vi "calibrate ESR.vi"(7 "Processing loop variables":T1 {"CurrInverter"."last updated" format="%<%H:%M\n%d/%m/%Y>T"; "CurrInverter"."set flag" items=["False", "True"]}, 8 "error in (no error)":errorcluster, 9 "Max ESR":dbl[](array[numeric]), 11 "Acquisition mode in":T8) -> (0 "error out":errorcluster, 3 "Processing loop vars out":T1 {"CurrInverter"."last updated" format="%<%H:%M\n%d/%m/%Y>T"; "CurrInverter"."set flag" items=["False", "True"]})   [LabVIEW 2019, in "Main.lvclass"]
uses:
  Main.lvclass
  Common/DataTypes/Acquisition Mode--cluster.ctl
  DataTypes/averaging variables.ctl
  DataTypes/ESR alarm variables.ctl
  Common/DataTypes/inverter gain range--cluster.ctl
  Common/DataTypes/inverter offset range--cluster.ctl
  Common/DataTypes/inverter info v2--cluster.ctl
  Common/DataTypes/Inverter database record v2--cluster.ctl
  DataTypes/Processing loop variables--cluster.ctl
panel:
  out "Calibration":dbl
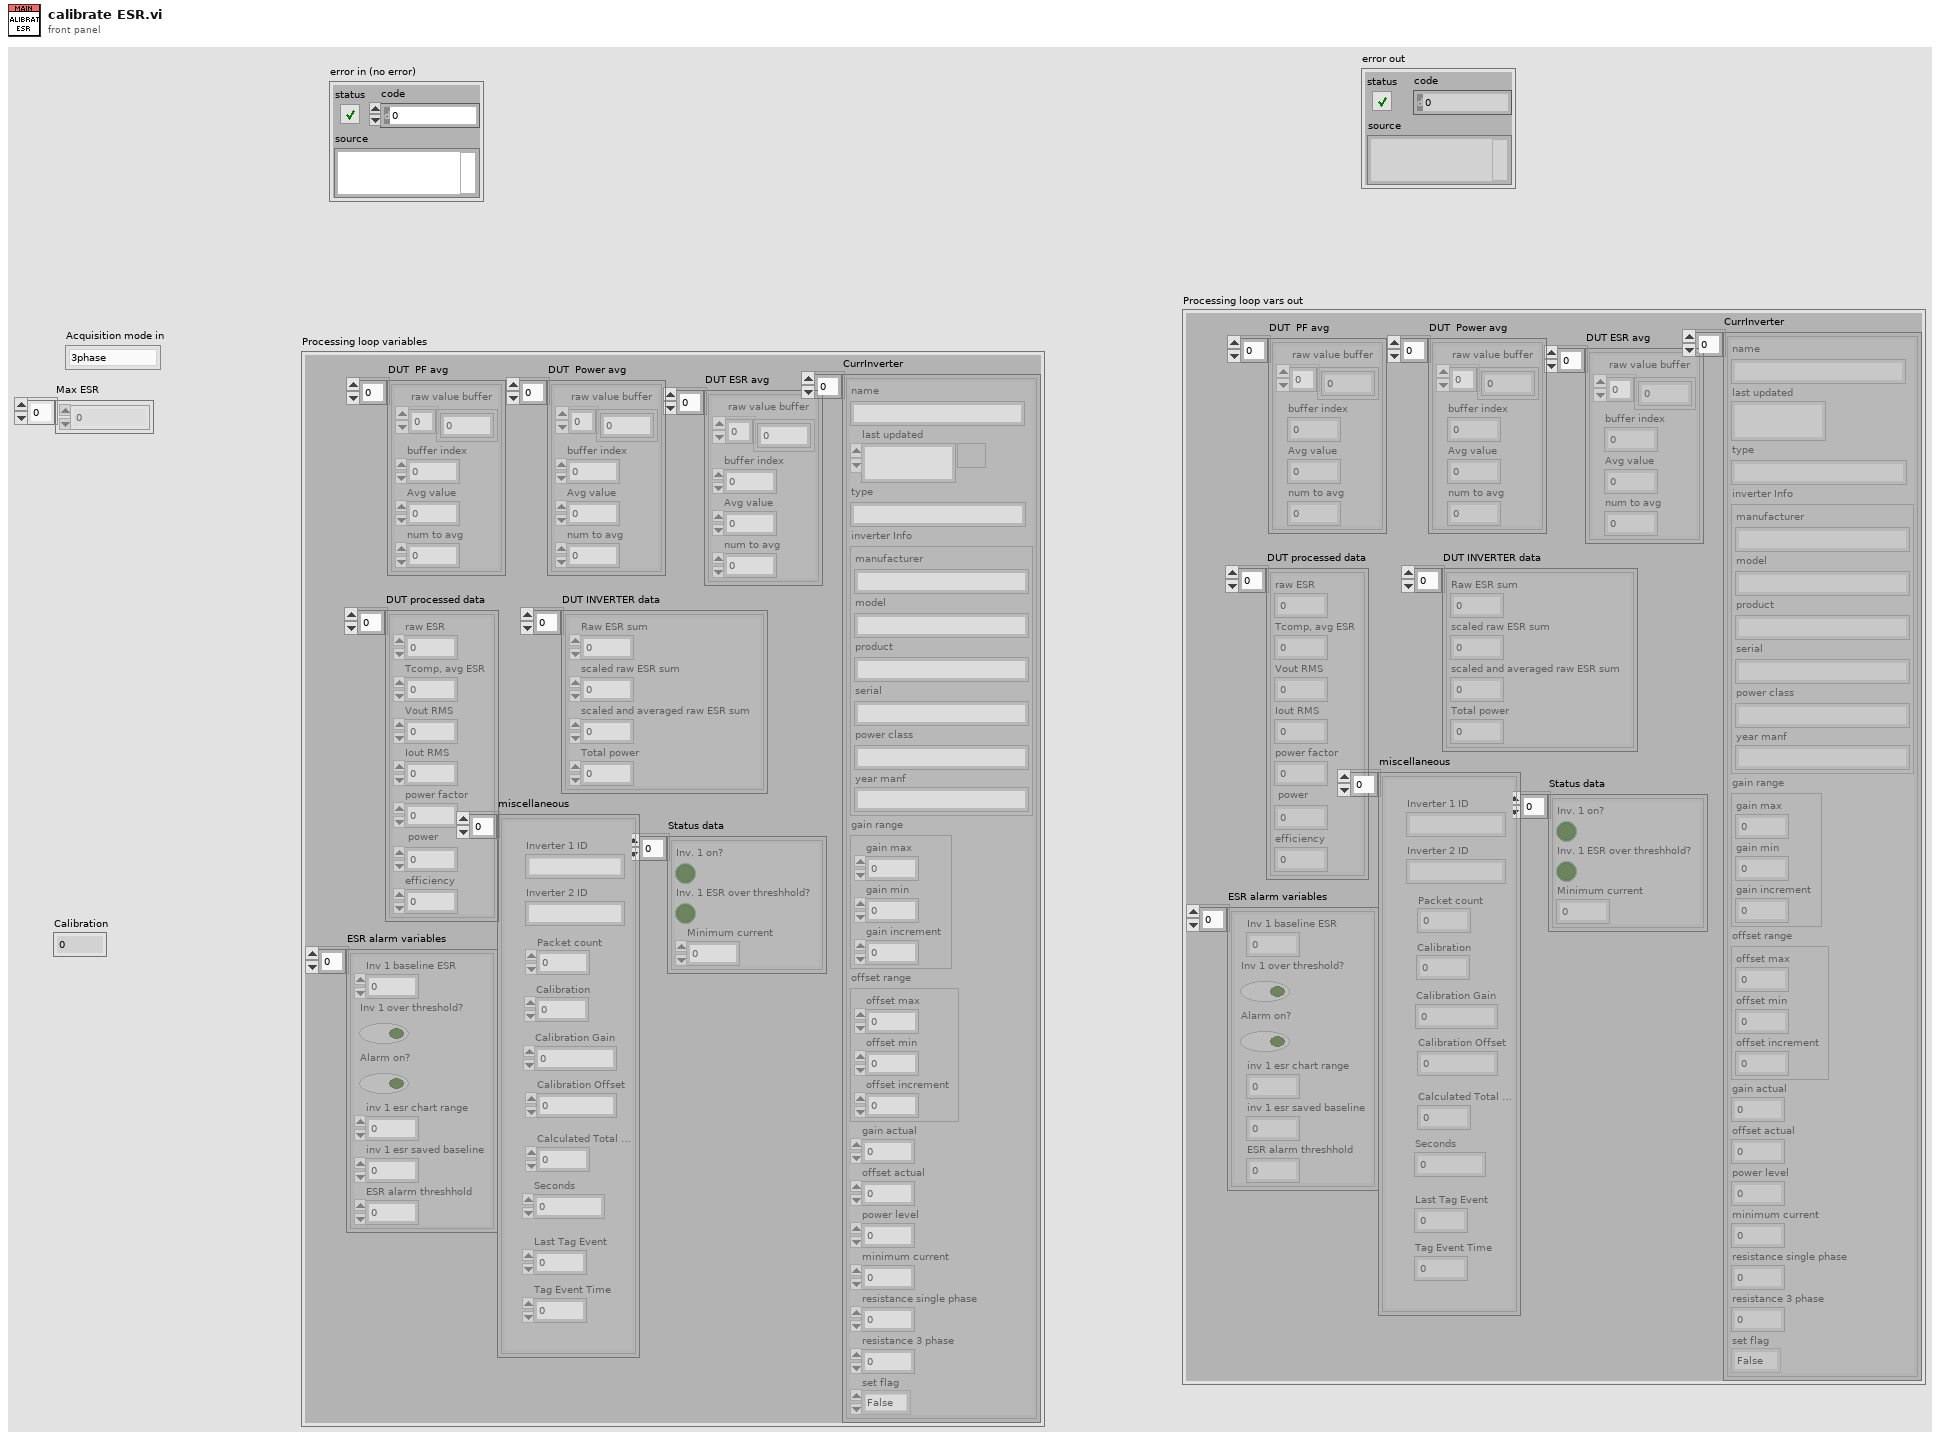
[diagram p1: front panel]
types:
  T1 = typedef "Main.lvclass/Processing loop variables--cluster.ctl" = cluster{"DUT ESR avg":T2[], "DUT  PF avg":T2[], "DUT  Power avg ":T2[], "DUT processed data":cluster{"raw ESR":dbl, "Tcomp, avg ESR":dbl, "Vout RMS":dbl, "Iout RMS":dbl, "power factor":dbl, "power":dbl, "efficiency":dbl}[], "ESR alarm variables":T3[], "Status data":cluster{"Inv. 1 on?":bool, "Inv. 1 ESR over threshhold?":bool, "Minimum current":dbl}[], "CurrInverter":T4[], "miscellaneous":cluster{"Inverter 1 ID":string, "Inverter 2 ID":string, "Packet count":u32, "Calibration":dbl, "Calibration Gain":dbl, "Calibration Offset":dbl, "Calculated Total Power":dbl, "Seconds":dbl, "Last Tag Event":dbl, "Tag Event Time":dbl}[], "DUT INVERTER data":cluster{"Raw ESR sum":dbl, "scaled raw ESR sum":dbl, "scaled and averaged raw ESR sum":dbl, "Total power":dbl}[]}
  T2 = typedef "Main.lvclass/averaging variables.ctl" = cluster{"raw value buffer":dbl[], "buffer index":i32, "Avg value":dbl, "num to avg":i32}
  T3 = typedef "Main.lvclass/ESR alarm variables.ctl" = cluster{"Inv 1 baseline ESR":dbl, "Inv 1 over threshold?":bool, "Alarm on?":bool, "inv 1 esr chart range":dbl, "inv 1 esr saved baseline":dbl, "ESR alarm threshhold":dbl}
  T4 = typedef "Inverter database record v2--cluster.ctl" = cluster{"name":string, "last updated":timestamp, "type":string, "inverter Info":T5, "gain range":T6, "offset range":T7, "gain actual":dbl, "offset actual":dbl, "power level":dbl, "minimum current":dbl, "resistance single phase":dbl, "resistance 3 phase":dbl, "set flag":u16}
  T5 = typedef "inverter info v2--cluster.ctl" = cluster{"manufacturer":string, "model":string, "product":string, "serial":string, "power class":string, "year manf":string}
  T6 = typedef "inverter gain range--cluster.ctl" = cluster{"gain max":dbl, "gain min":dbl, "gain increment":dbl}
  T7 = typedef "inverter offset range--cluster.ctl" = cluster{"offset max":dbl, "offset min":dbl, "offset increment":dbl}
  T8 = typedef "Acquisition Mode--cluster.ctl" = enum16{"3phase", "Single"}
  T9 = cluster{"Inverter 1 ID":string, "Inverter 2 ID":string, "Packet count":u32, "Calibration":dbl, "Calibration Gain":dbl, "Calibration Offset":dbl, "Calculated Total Power":dbl, "Seconds":dbl, "Last Tag Event":dbl, "Tag Event Time":dbl}[]
  T10 = cluster{"Raw ESR sum":dbl, "scaled raw ESR sum":dbl, "scaled and averaged raw ESR sum":dbl, "Total power":dbl}[]
  T11 = cluster{"Inverter 1 ID":string, "Inverter 2 ID":string, "Packet count":u32, "Calibration":dbl, "Calibration Gain":dbl, "Calibration Offset":dbl, "Calculated Total Power":dbl, "Seconds":dbl, "Last Tag Event":dbl, "Tag Event Time":dbl}
  T12 = cluster{string, "time string":string, "t":dbl, "Calibration Gain":dbl, "Calibration Offset":dbl, "Max ESR":dbl, "Acquisition mode in":T8, "name":string, "serial":string, "Total power":dbl}
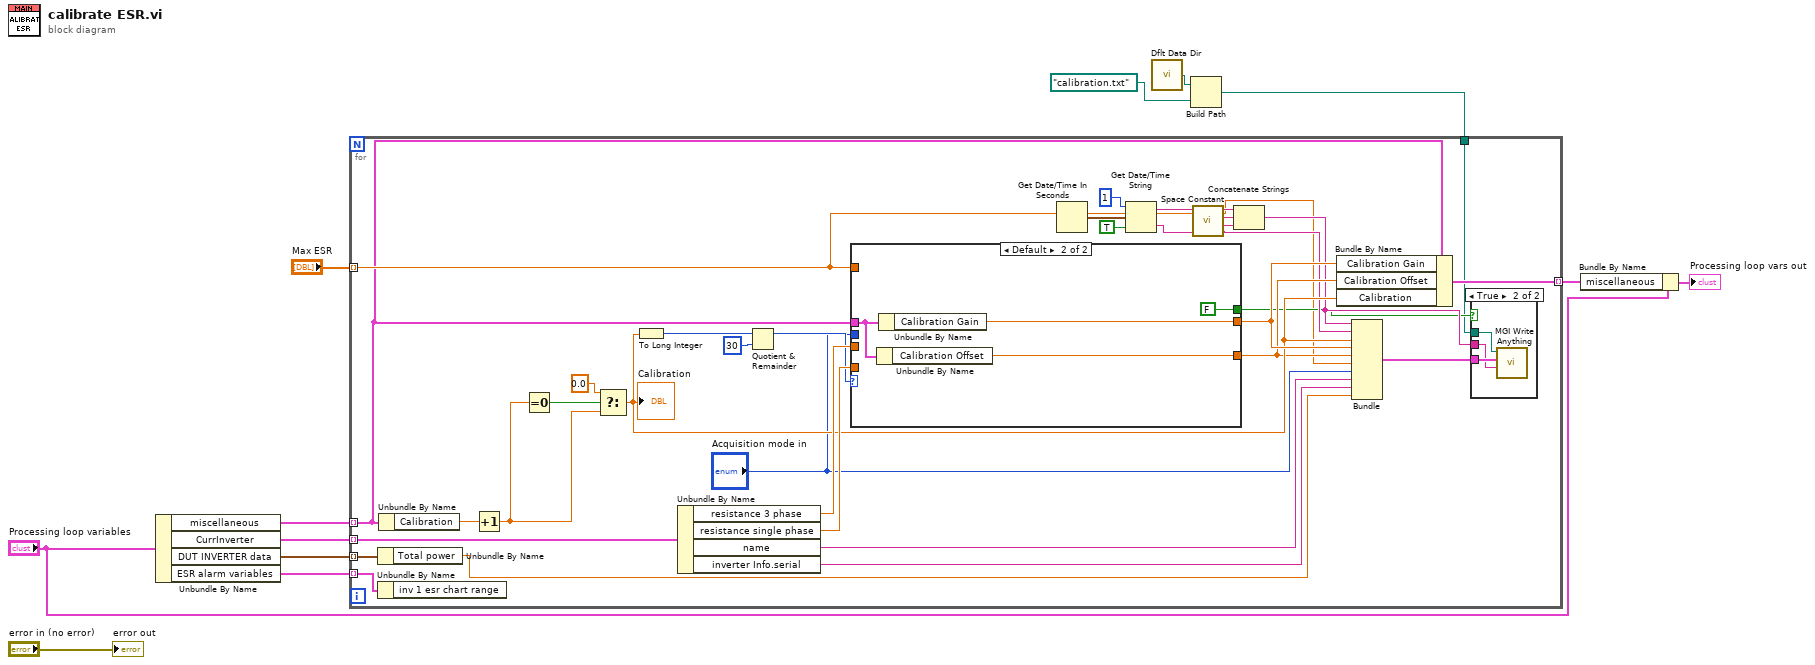
[diagram p0: block diagram]
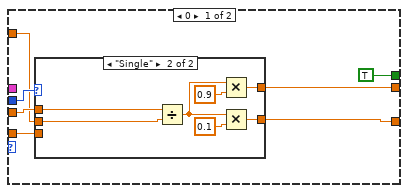
[diagram p3: hidden frame]
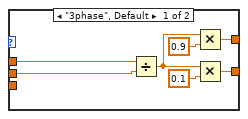
[diagram p4: hidden frame]
diagram:
  n1 = Unbundle By Name("Processing loop variables") -> ("miscellaneous"=w11:T9, "CurrInverter"=w10:T4[], "DUT INVERTER data"=w9:T10, "ESR alarm variables"=w5:T3[])
  n2 = call <vilib>:"Dflt Data Dir.vi"() -> ("App:Default Data Directory"=w3:path)
  n3 = Build Path(base path=w3, name or relative path=path "calibration.txt") -> (appended path=w1:path)
  n4 = for {
    tunnel: w11 -> [w14] mode=indexing
    tunnel: w10 -> [w44] mode=indexing
    tunnel: w9 -> [w43] mode=indexing
    tunnel: [w42] -> w6 mode=indexing
    tunnel: w5 -> [w16] mode=indexing
    tunnel: "Max ESR" -> [w15] mode=indexing
    tunnel: w1 -> [w13]
    n5 = Unbundle By Name(w43) -> ("Total power"=w17:dbl)
    n6 = Unbundle By Name(w16) -> ()  [unwired: 1 out]
    n7 = Unbundle By Name(w14) -> ("Calibration"=w40:dbl)
    n8 = Increment(x=w40) -> (x+1=w36:dbl)
    n9 = Equal To 0?(x=w36) -> (x = 0?=w34:bool)
    n10 = Select(t=0.0, s=w34, f=w36) -> (s? t:f=w30:dbl)
    "Calibration" <- w30
    n11 = To Long Integer(number=w30) -> (32bit integer=w32:i32)
    n12 = Unbundle By Name(w44) -> ("resistance 3 phase"=w41:dbl, "resistance single phase"=w39:dbl, "name"=w22:string, "inverter Info.serial"=w21:string)
    n13 = Quotient & Remainder(x=w32, y=30) -> (x-y*floor(x/y)=w31:i32)  [unwired: 1 out]
    n14 = case shown="Default" w31 {
      tunnel: "Acquisition mode in" -> [w54 _]
      tunnel: w41 -> [w53 _]
      tunnel: w15 -> [w52 _]
      tunnel: w39 -> [w51 _]
      tunnel: [w50 w72] -> w38
      tunnel: [w49 w70] -> w28
      tunnel: w14 -> [_ w71]
      tunnel: [TRUE FALSE] -> w18
      frame 0 {
        n15 = case shown="\"Single\"" w54 {
          tunnel: w53 -> [w59 w64]
          tunnel: w52 -> [w61 w63]
          tunnel: [w57 w66] -> w49
          tunnel: [w55 w62] -> w50
          tunnel: w51 -> [_ _]
          frame "3phase", Default {
            n16 = Divide(x=w59, y=w61) -> (x/y=w58:dbl)
            n17 = Multiply(x=w58, y=0.9) -> (x*y=w55:dbl)
            n18 = Multiply(x=w58, y=0.1) -> (x*y=w57:dbl)
          }
          frame "Single" {
            n19 = Divide(x=w64, y=w63) -> (x/y=w68:dbl)
            n20 = Multiply(x=w68, y=0.9) -> (x*y=w62:dbl)
            n21 = Multiply(x=w68, y=0.1) -> (x*y=w66:dbl)
          }
        }
      }
      frame Default {
        n22 = Unbundle By Name(w71) -> ("Calibration Offset"=w70:dbl)
        n23 = Unbundle By Name(w71) -> ("Calibration Gain"=w72:dbl)
      }
    }
    n24 = Get Date/Time In Seconds() -> (seconds since 1Jan1904=w29:timestamp)
    n25 = Get Date/Time String(date format (0)=1, seconds (now)=w29, want seconds? (F)=TRUE) -> (date string=w27:string, time string=w20:string)
    n26 = call <vilib>:"Space Constant.vi"() -> ("String"=w24:string)
    n27 = Concatenate Strings(w27, w24, w20) -> (w26:string)
    n28 = Bundle By Name(cluster=w14, "Calibration Gain"=w38, "Calibration Offset"=w28, "Calibration"=w30) -> (w42:T11)
    n29 = Bundle(w26, "time string"=w20, "t"=w30, "Calibration Gain"=w38, "Calibration Offset"=w28, "Max ESR"=w15, "Acquisition mode in"="Acquisition mode in", "name"=w22, "serial"=w21, "Total power"=w17) -> (w37:T12)  [unwired: 1 in]
    n30 = case shown="True" w18 {
      tunnel: w37 -> [_ w47]
      tunnel: w13 -> [_ w46]
      tunnel: w26 -> [_ w45]
      frame False {
      }
      frame True {
        n31 = call <userlib>:"MGI Write Anything.vi"("Section Name (Name of \"Anything\")"=w45, "Anything"=w47, "Path (dialog)"=w46) -> ()  [unwired: 6 in, 3 out]
      }
    }
  }
  n32 = Bundle By Name(cluster="Processing loop variables", "miscellaneous"=w6) -> (→"Processing loop vars out":T1)
  "error out" <- "error in (no error)"
